vi "Write NPort 1Samp 1D Boolean.vi"(8 "error in (no error)":errorcluster, 9 "values":u8[](array[numeric]) format="%08b", 10 "Ports (Banks)":T1[](array[typedef]) items=["DIO1...8"=1, "DIO9...16"=2, "DIO17...24"=3, "DIO25...32"=4], 11 "MicroDAQ.lvlib:Digital output.lvclass":refnum<class "Digital output.lvclass">) -> (0 "error out":errorcluster, 3 "MicroDAQ.lvlib:Digital output.lvclass out":refnum<class "Digital output.lvclass">)   [LabVIEW 2009, in "MicroDAQ.lvlib" / "Digital output.lvclass"]
doc: "Writes a array of U8 registers to a digital output channel composed of a multiple ports."
uses:
  <instrlib>/MicroDAQ/Channel/Digital output/Digital output.lvclass
  <instrlib>/MicroDAQ/Tools/Digital IO channels.ctl
  <instrlib>/MicroDAQ/MicroDAQ.lvlib
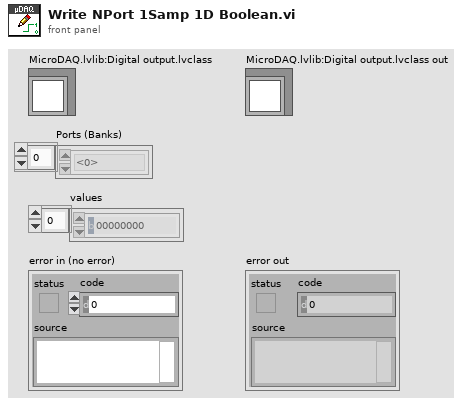
[diagram p1: front panel]
types:
  T1 = typedef "MicroDAQ.lvlib/Digital IO channels.ctl" = u8
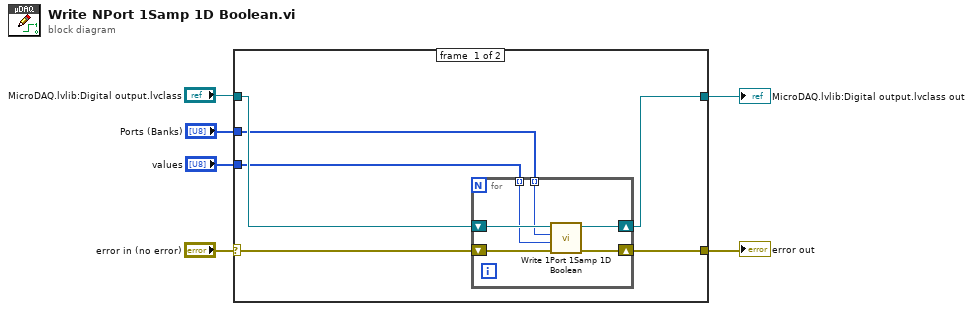
[diagram p0: block diagram]
diagram:
  n1 = case shown="No Error" "error in (no error)" {
    selector: "error in (no error)" -> [w12 w19]
    tunnel: [w11 w19] -> w5
    tunnel: "MicroDAQ.lvlib:Digital output.lvclass" -> [w10 w20]
    tunnel: [w9 w20] -> w3
    tunnel: "Ports (Banks)" -> [w8 _]
    tunnel: "values" -> [w7 _]
    frame #0 {
      n2 = for {
        shift-right: [w17] -> w11
        shift-left: w12 -> [w18]
        shift-right: [w15] -> w9
        shift-left: w10 -> [w16]
        tunnel: w8 -> [w14] mode=indexing
        tunnel: w7 -> [w13] mode=indexing
        n3 = call <instrlib>:"Write 1Port 1Samp 1D Boolean.vi"("error in (no error)"=w18, "value"=w13, "Port (Bank)"=w14, "MicroDAQ.lvlib:Digital output.lvclass"=w16) -> ("error out"=w17:errorcluster, "MicroDAQ.lvlib:Digital output.lvclass out"=w15:refnum<class "Digital output.lvclass">)  [unwired: 6 in]
      }
    }
    frame #1 {
    }
  }
  "error out" <- w5
  "MicroDAQ.lvlib:Digital output.lvclass out" <- w3
